vi "MathNode.vi"() -> ()   [LabVIEW 2022 SP3]
uses:
  <vilib>/numeric/Random Number (Range) U64.vi
  <vilib>/numeric/sub_Random U32.vi
panel:
  out "T2 in °C":dbl[](array[numeric])
  in  "Constant B":dbl
  in  "Constant A":dbl
  out "T1 in °C":dbl[](array[numeric])
  in  "# Of random Numbers":i32
  out "Array":u64[](array[numeric])
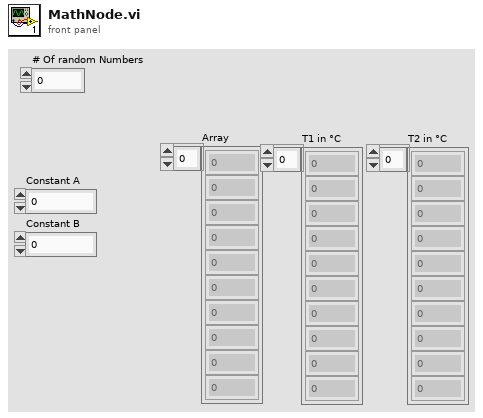
[diagram p1: front panel]
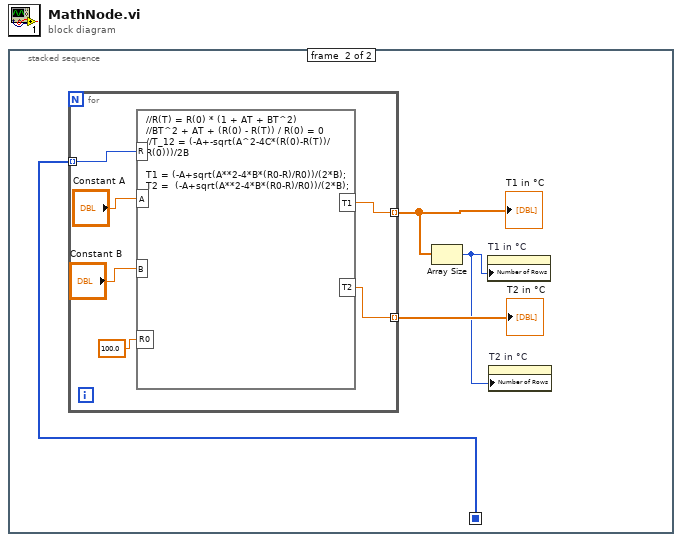
[diagram p0: block diagram]
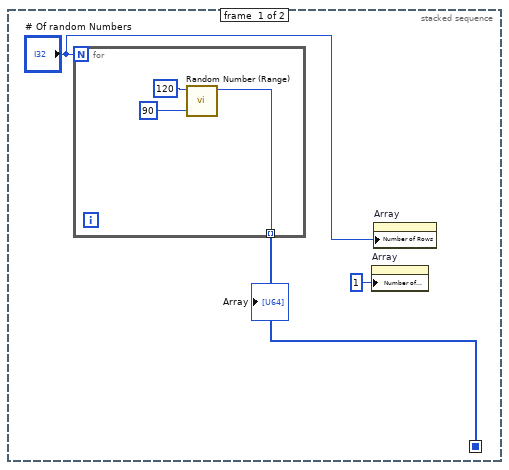
[diagram p2: hidden frame]
diagram:
  n1 = stacked-sequence {
    seq-local: [w3 _] -> [_ w10]
    frame #0 {
      n2 = for {
        N: "# Of random Numbers" -> [_]
        tunnel: [w4] -> w3 mode=indexing
        n3 = call-poly <vilib>:"Random Number (Range).vi"("lower bound (0)"=u64 90, "upper bound (100)"=u64 120) -> ("number"=w4:u64)  [unwired: 9 in]
      }
      "Array" <- w3
      n4 = property on="Array" class="Arr (strict)"("Number of Columns"=u32 1) -> ()  [unwired: 2 in, 2 out]
      n5 = property on="Array" class="Arr (strict)"("Number of Rows"="# Of random Numbers") -> ()  [unwired: 2 in, 2 out]
    }
    frame #1 {
      n6 = for {
        tunnel: w10 -> [w16] mode=indexing
        tunnel: [w15] -> w9 mode=indexing
        tunnel: [w11] -> w8 mode=indexing
        n7 = formula code="//R(T) = R(0) * (1 + AT + BT^2)\n//BT^2 + AT + (R(0) - R(T)) / R(0) = 0\n//T_12 = (-A+-sqrt(A^2-4C*(R(0)-R(T))/R(0)))/2B\n\nT1 = (-A+sqrt(A**2-4*B*(R0-R)/R0))/(2*B);\nT2 =  (-A+sqrt(A**2-4*B*(R0-R)/R0))/(2*B);"("R"=w16, "A"="Constant A", "B"="Constant B", "R0"=100.0 ("input variable")) -> ("T1"=w15:dbl, "T2"=w11:dbl)
      }
      "T1 in °C" <- w9
      "T2 in °C" <- w8
      n8 = Array Size(array=w9) -> (size(s)=w7:i32)
      n9 = property on="T1 in °C" class="Arr (strict)"("Number of Rows"=w7) -> ()  [unwired: 2 in, 2 out]
      n10 = property on="T2 in °C" class="Arr (strict)"("Number of Rows"=w7) -> ()  [unwired: 2 in, 2 out]
    }
  }
